vi "p2.vi"() -> ()   [LabVIEW 2025, in "d9.lvlib"]
uses:
  d9.lvlib
  <vilib>/Analysis/geometry.llb/Point in Polygon Position.ctl
  f819d5f4-ec59-4299-be88-67458834ba28.vi
  <vilib>/Analysis/geometry.llb/Point in Polygon (Array).vi
  <vilib>/Comparison/Less/Less Functor/Less Functor.lvclass
  AOC/AOC.lvlib
  <vilib>/Analysis/NI_AAL_Geometry.lvlib
panel:
  out "red tile 2":T1
  out "red tile 1":T1
  out "Floor Plan":T2(graph)
  out "Area 2":u64
  in  "Example":string="7,1\n11,1\n11,7\n9,7\n9,5\n2,5\n2,3\n7,3"
  in  "Example 2":bool
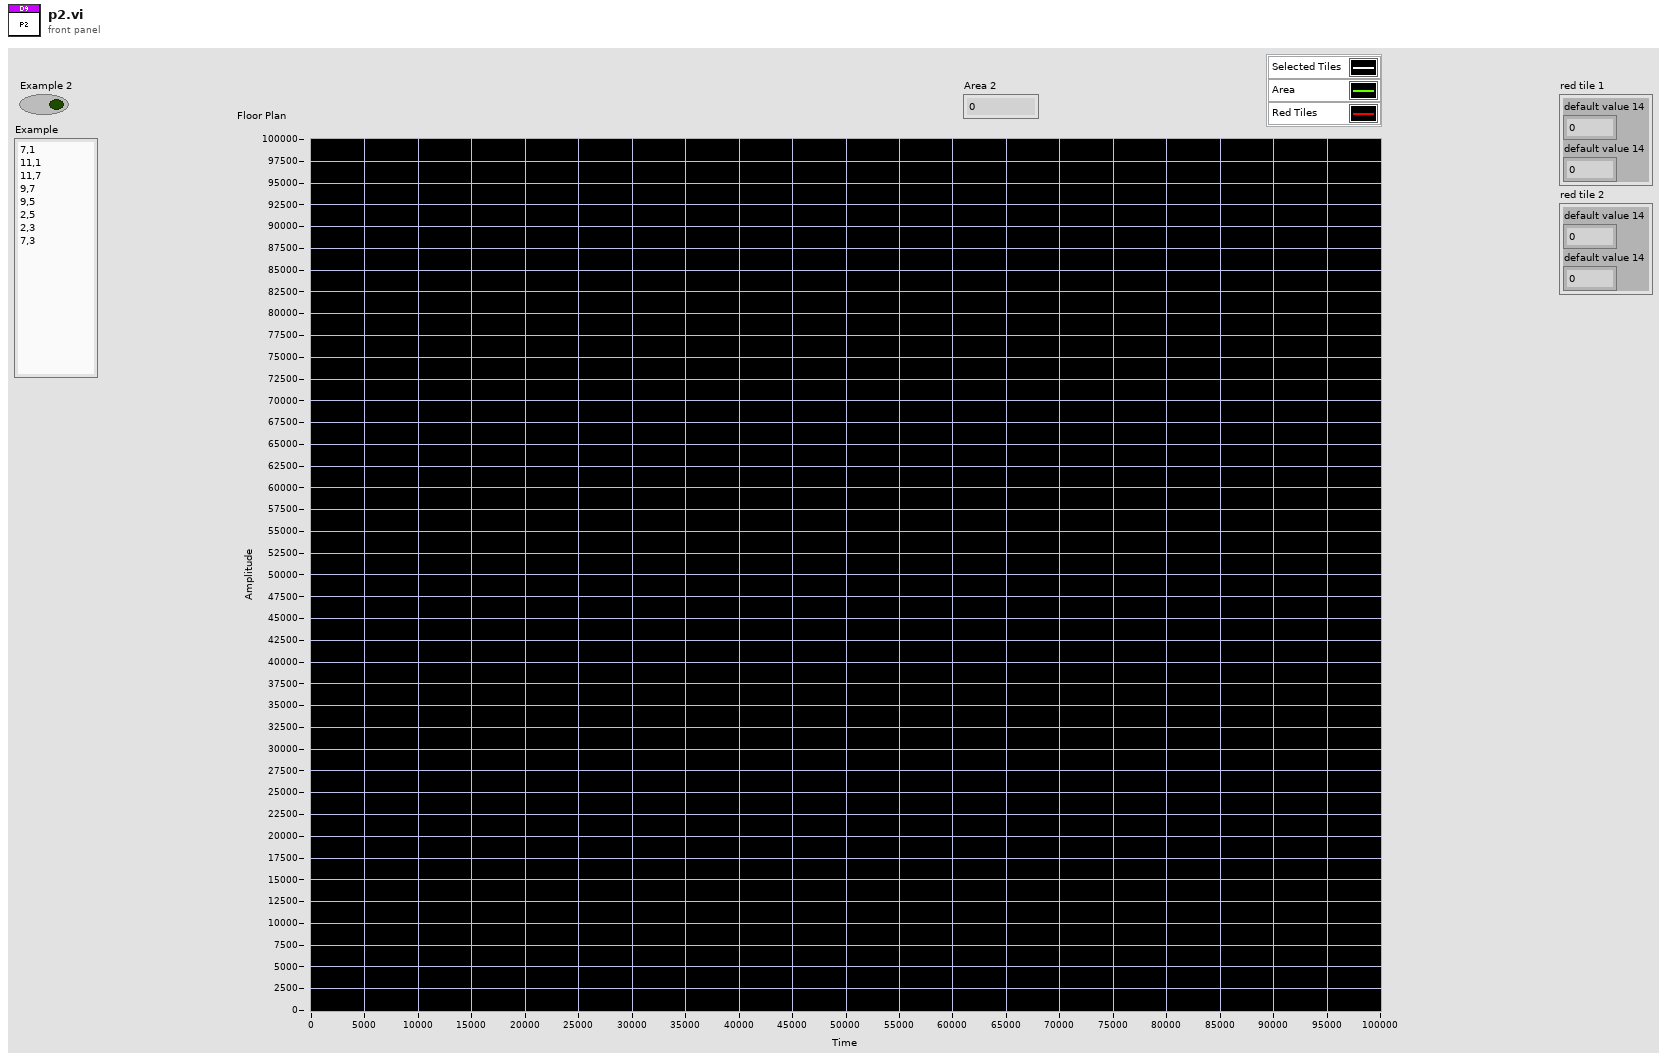
[diagram p1: front panel]
types:
  T1 = cluster{"default value 14":i64, "default value 14":i64}
  T2 = cluster{cluster{"default value 14":i64, "default value 14":i64}[]}[]
  T3 = cluster{"default value 14":i64, "default value 14":i64}[]
  T4 = typedef "NI_AAL_Geometry.lvlib/Point in Polygon Position.ctl" = u16
  T5 = cluster{cluster{"default value 14":i64, "default value 14":i64}[]}
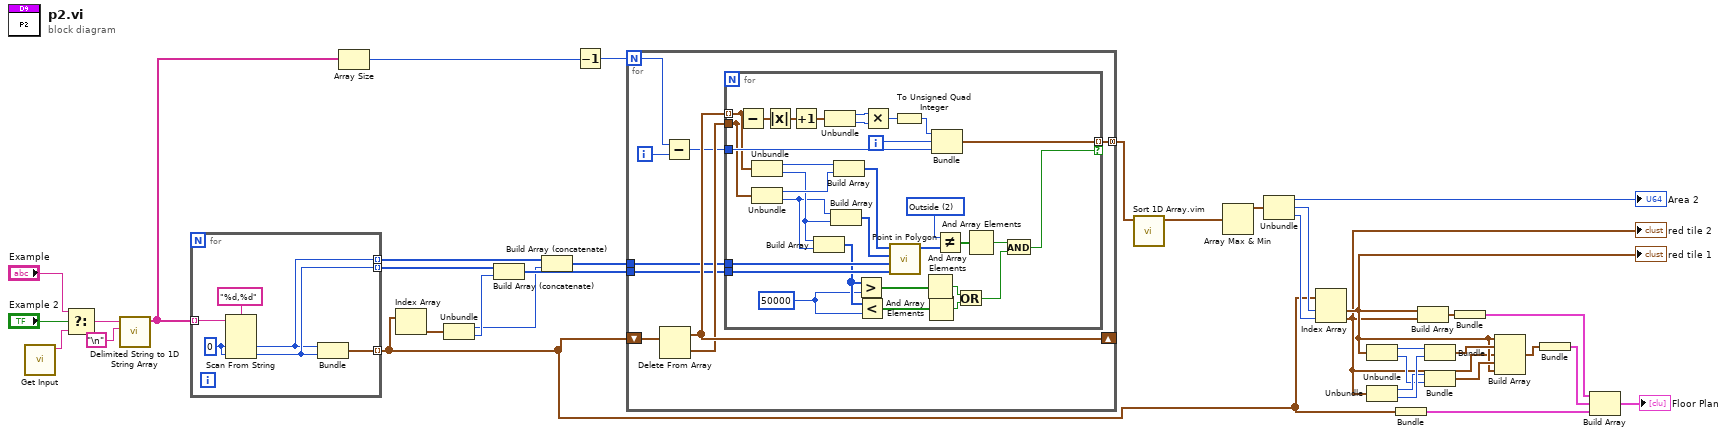
[diagram p0: block diagram]
diagram:
  n1 = call "Get Input.vi"() -> ("Input"=w34:string)  [unwired: 11 in]
  n2 = Select(t="Example", s="Example 2", f=w34) -> (s? t:f=w31:string)
  n3 = call <vilib>:"Delimited String to 1D String Array.vi"("delimiter"="\n", "delimited string"=w31) -> ("string array"=w26:string[])  [unwired: 9 in]
  n4 = for {
    tunnel: w26 -> [w42] mode=indexing
    tunnel: [w39] -> w2 mode=indexing
    tunnel: [w38] -> w29 mode=indexing
    tunnel: [w37] -> w25 mode=indexing
    w40 = i64 0 ("default value 14")
    n5 = Scan From String(format string="%d,%d", input string=w42, default 1=w40, default 2=w40) -> (output 1=w37:i64, output 2=w38:i64)  [unwired: 2 in, 3 out]
    n6 = Bundle("default value 14"=w37, "default value 14"=w38) -> (w39:T1)  [unwired: 1 in]
  }
  n7 = Array Size(array=w26) -> (size(s)=w32:i32)
  n8 = Index Array(array=w2) -> (element=w24:T1)  [unwired: 1 in]
  n9 = Unbundle(w24) -> ("default value 14"=w22:i64, "default value 14"=w23:i64)
  n10 = Build Array (concatenate)(w29, w23) -> (w27:i64[])
  n11 = Build Array (concatenate)(w25, w22) -> (w28:i64[])
  n12 = Decrement(x=w32) -> (x-1=w30:i32)
  n13 = for {
    N: w30 -> [w45]
    shift-right: [w50] -> _
    shift-left: w2 -> [w51]
    tunnel: [w48] -> w3 mode=concatenating
    tunnel: w28 -> [w44]
    tunnel: w27 -> [w43]
    i -> [w46]
    n14 = Delete From Array(array=w51) -> (deleted portion=w49:T1, array with subset deleted=w50:T3)  [unwired: 2 in]
    n15 = Subtract(x=w45, y=w46) -> (x-y=w47:i32)
    n16 = for {
      tunnel: w50 -> [w73] mode=indexing
      tunnel: w49 -> [w72]
      tunnel: w47 -> [w77]
      tunnel: [w76] -> w48 mode=indexing if=w52
      tunnel: w44 -> [w71]
      tunnel: w43 -> [w70]
      i -> [w78]
      w59 = i64 50000 ("y")
      w68 = T4 2 items=["Inside", "On Boundary", "Outside"] ("x")
      n17 = Subtract(x=w73, y=w72) -> (x-y=w83:T1)
      n18 = Unbundle(w73) -> ("default value 14"=w65:i64, "default value 14"=w62:i64)
      n19 = Unbundle(w72) -> ("default value 14"=w66:i64, "default value 14"=w61:i64)
      n20 = Absolute Value(x=w83) -> (abs(x)=w82:T1)
      n21 = Increment(x=w82) -> (x+1=w74:T1)
      n22 = Build Array(w62, w61) -> (w60:i64[])
      n23 = Unbundle(w74) -> ("default value 14"=w81:i64, "default value 14"=w80:i64)
      n24 = Build Array(w61, w62) -> (w63:i64[])
      n25 = Build Array(w65, w66) -> (w64:i64[])
      n26 = Greater?(x=w60, y=w59) -> (0:w58:bool[])
      n27 = Less?(x=w60, y=w59) -> (x < y?=w57:bool[])
      n28 = Multiply(x=w81, y=w80) -> (x*y=w79:i64)
      n29 = call-poly <vilib>:"Point in Polygon.vi"("Polygon Y"=w70, "Polygon X"=w71, "Y"=w63, "X"=w64) -> ("Position"=w69:T4[])  [unwired: 6 in, 1 out]
      n30 = To Unsigned Quad Integer(1:w79) -> (0:w75:u64)
      n31 = And Array Elements(Boolean array=w58) -> (logical AND=w55:bool)
      n32 = And Array Elements(Boolean array=w57) -> (logical AND=w56:bool)
      n33 = Bundle(w75, w78, w77) -> (w76:cluster{u64, i32, i32})  [unwired: 1 in]
      n34 = Not Equal?(x=w68, y=w69) -> (x != y?=w67:bool[])
      n35 = Or(x=w55, y=w56) -> (x .or. y?=w53:bool)
      n36 = And Array Elements(Boolean array=w67) -> (logical AND=w54:bool)
      n37 = And(x=w54, y=w53) -> (x .and. y?=w52:bool)
    }
  }
  n38 = call "Sort 1D Array.vim"("unsorted array"=w3) -> ("sorted array"=w1:cluster{u64, i32, i32}[])  [unwired: 10 in]
  n39 = Array Max & Min(array=w1) -> (max value=w21:cluster{u64, i32, i32})  [unwired: 3 out]
  n40 = Unbundle(w21) -> (→"Area 2":u64, w20:i32, w18:i32)
  n41 = Index Array(array=w2, index #1=w20, index #2=w18) -> (element #1=w5:T1, element #2=w4:T1)
  "red tile 1" <- w5
  "red tile 2" <- w4
  n42 = Unbundle(w5) -> ("default value 14"=w13:i64, "default value 14"=w7:i64)
  n43 = Unbundle(w4) -> ("default value 14"=w8:i64, "default value 14"=w12:i64)
  n44 = Bundle(w2) -> (w17:T5)  [unwired: 1 in]
  n45 = Build Array(w5, w4) -> (w15:T3)
  n46 = Bundle("default value 14"=w13, "default value 14"=w12) -> (w11:T1)  [unwired: 1 in]
  n47 = Bundle("default value 14"=w8, "default value 14"=w7) -> (w6:T1)  [unwired: 1 in]
  n48 = Bundle(w15) -> (w14:T5)  [unwired: 1 in]
  n49 = Build Array(w5, w11, w4, w6, w5) -> (w9:T3)
  n50 = Bundle(w9) -> (w10:T5)  [unwired: 1 in]
  n51 = Build Array(w14, w10, w17) -> (→"Floor Plan":T2)
